vi "GeoData.vi"() -> ()   [LabVIEW 2017] (continued)
H1\n85013\t4013\tPhoenix\tAZ\tMaricopa County\tH1\n85018\t4013\tPhoenix\tAZ\tMaricopa County\tH1\n85301\t4013\tGlendale\tAZ\tMaricopa County\tH1\n85298\t4013\tGilbert\tAZ\tMaricopa County\tH1\n85338\t4013\tGoodyear\tAZ\tMaricopa County\tH1\n85353\t4013\tTolleson\tAZ\tMaricopa County\tH1\n85378\t4013\tSurprise\tAZ\tMaricopa County\tH1\n85064\t4013\tPhoenix\tAZ\tMaricopa County\tH1\n85002\t4013\tPhoenix\tAZ\tMaricopa County\tH1\n85377\t4013\tCarefree\tAZ\tMaricopa County\tH1\n85322\t4013\tArlington\tAZ\tMaricopa County\tH1\n85010\t4013\tPhoenix\tAZ\tMaricopa County\tH1\n85033\t4013\tPhoenix\tAZ\tMaricopa County\tH1\n85041\t4013\tPhoenix\tAZ\tMaricopa County\tH1\n85050\t4013\tPhoenix\tAZ\tMaricopa County\tH1\n85046\t4013\tPhoenix\tAZ\tMaricopa County\tH1\n85080\t4013\tPhoenix\tAZ\tMaricopa County\tH1\n85078\t4013\tPhoenix\tAZ\tMaricopa County\tH1\n85143\t4013\tSan tan valley\tAZ\tMaricopa County\tH1\n85209\t4013\tMesa\tAZ\tMaricopa County\tH1\n85213\t4013\tMesa\tAZ\tMaricopa County\tH1\n85250\t4013\tScottsdale\tAZ\tMaricopa County\tH1\n85261\t4013\tScottsdale\tAZ\tMaricopa County\tH1\n85007\t4013\tPhoenix\tAZ\tMaricopa County\tH1\n85012\t4013\tPhoenix\tAZ\tMaricopa County\tH1\n85015\t4013\tPhoenix\tAZ\tMaricopa County\tH1\n85306\t4013\tGlendale\tAZ\tMaricopa County\tH1\n85335\t4013\tEl mirage\tAZ\tMaricopa County\tH1\n85354\t4013\tTonopah\tAZ\tMaricopa County\tH1\n85339\t4013\tLaveen\tAZ\tMaricopa County\tH1\n85383\t4013\tPeoria\tAZ\tMaricopa County\tH1\n85274\t4013\tMesa\tAZ\tMaricopa County\tH1\n85069\t4013\tPhoenix\tAZ\tMaricopa County\tH1\n85385\t4013\tPeoria\tAZ\tMaricopa County\tH1\n85036\t4013\tPhoenix\tAZ\tMaricopa County\tH1\n85071\t4013\tPhoenix\tAZ\tMaricopa County\tH1\n85127\t4013\tChandler heights\tAZ\tMaricopa County\tH1\n85372\t4013\tSun city\tAZ\tMaricopa County\tH1\n85287\t4013\tTempe\tAZ\tMaricopa County\tH1\n86442\t4015\tBullhead city\tAZ\tMohave County\tH1\n86429\t4015\tBullhead city\tAZ\tMohave County\tH1\n86430\t4015\tBullhead city\tAZ\tMohave County\tH1\n86443\t4015\tTemple bar marina\tAZ\tMohave County\tH1\n86401\t4015\tKingman\tAZ\tMohave County\tH1\n86413\t4015\tGolden valley\tAZ\tMohave County\tH1\n86402\t4015\tKingman\tAZ\tMohave County\tH1\n86445\t4015\tWillow beach\tAZ\tMohave County\tH1\n85360\t4015\tWikieup\tAZ\tMohave County\tH1\n86404\t4015\tLake havasu city\tAZ\tMohave County\tH1\n86426\t4015\tFort mohave\tAZ\tMohave County\tH1\n86411\t4015\tHackberry\tAZ\tMohave County\tH1\n86021\t4015\tColorado city\tAZ\tMohave County\tH1\n86440\t4015\tMohave valley\tAZ\tMohave County\tH1\n86434\t4015\tPeach springs\tAZ\tMohave County\tH1\n86446\t4015\tMohave valley\tAZ\tMohave County\tH1\n86431\t4015\tChloride\tAZ\tMohave County\tH1\n86403\t4015\tLake havasu city\tAZ\tMohave County\tH1\n86406\t4015\tLake havasu city\tAZ\tMohave County\tH1\n86441\t4015\tDolan springs\tAZ\tMohave County\tH1\n86436\t4015\tTopock\tAZ\tMohave County\tH1\n86438\t4015\tYucca\tAZ\tMohave County\tH1\n86409\t4015\tKingman\tAZ\tMohave County\tH1\n86412\t4015\tHualapai\tAZ\tMohave County\tH1\n86437\t4015\tValentine\tAZ\tMohave County\tH1\n86439\t4015\tBullhead city\tAZ\tMohave County\tH1\n86432\t4015\tLittlefield\tAZ\tMohave County\tH1\n86444\t4015\tMeadview\tAZ\tMohave County\tH1\n86405\t4015\tLake havasu city\tAZ\tMohave County\tH1\n86427\t4015\tFort mohave\tAZ\tMohave County\tH1\n86433\t4015\tOatman\tAZ\tMohave County\tH1\n85942\t4017\tWoodruff\tAZ\tNavajo County\tH1\n86520\t4017\tBlue gap\tAZ\tNavajo County\tH1\n85935\t4017\tPinetop\tAZ\tNavajo County\tH1\n85901\t4017\tShow low\tAZ\tNavajo County\tH1\n86043\t4017\tSecond mesa\tAZ\tNavajo County\tH1\n85929\t4017\tLakeside\tAZ\tNavajo County\tH1\n86047\t4017\tWinslow\tAZ\tNavajo County\tH1\n86034\t4017\tKeams canyon\tAZ\tNavajo County\tH1\n85902\t4017\tShow low\tAZ\tNavajo County\tH1\n86039\t4017\tKykotsmovi village\tAZ\tNavajo County\tH1\n85926\t4017\tFort apache\tAZ\tNavajo County\tH1\n86029\t4017\tSun valley\tAZ\tNavajo County\tH1\n85928\t4017\tHeber\tAZ\tNavajo County\tH1\n86025\t4017\tHolbrook\tAZ\tNavajo County\tH1\n85933\t4017\tOvergaard\tAZ\tNavajo County\tH1\n85923\t4017\tClay springs\tAZ\tNavajo County\tH1\n85911\t4017\tCibecue\tAZ\tNavajo County\tH1\n86054\t4017\tShonto\tAZ\tNavajo County\tH1\n85937\t4017\tSnowflake\tAZ\tNavajo County\tH1\n86033\t4017\tKayenta\tAZ\tNavajo County\tH1\n86510\t4017\tPinon\tAZ\tNavajo County\tH1\n86042\t4017\tPolacca\tAZ\tNavajo County\tH1\n85939\t4017\tTaylor\tAZ\tNavajo County\tH1\n85941\t4017\tWhiteriver\tAZ\tNavajo County\tH1\n85934\t4017\tPinedale\tAZ\tNavajo County\tH1\n86031\t4017\tIndian wells\tAZ\tNavajo County\tH1\n86032\t4017\tJoseph city\tAZ\tNavajo County\tH1\n86030\t4017\tHotevilla\tAZ\tNavajo County\tH1\n85730\t4019\tTucson\tAZ\tPima County\tH1\n85740\t4019\tTucson\tAZ\tPima County\tH1\n85754\t4019\tTucson\tAZ\tPima County\tH1\n85724\t4019\tTucson\tAZ\tPima County\tH1\n85321\t4019\tAjo\tAZ\tPima County\tH1\n85736\t4019\tTucson\tAZ\tPima County\tH1\n85747\t4019\tTucson\tAZ\tPima County\tH1\n85714\t4019\tTucson\tAZ\tPima County\tH1\n85756\t4019\tTucson\tAZ\tPima County\tH1\n85658\t4019\tMarana\tAZ\tPima County\tH1\n85701\t4019\tTucson\tAZ\tPima County\tH1\n85645\t4019\tAmado\tAZ\tPima County\tH1\n85726\t4019\tTucson\tAZ\tPima County\tH1\n85743\t4019\tTucson\tAZ\tPima County\tH1\n85745\t4019\tTucson\tAZ\tPima County\tH1\n85746\t4019\tTucson\tAZ\tPima County\tH1\n85735\t4019\tTucson\tAZ\tPima County\tH1\n85733\t4019\tTucson\tAZ\tPima County\tH1\n85704\t4019\tTucson\tAZ\tPima County\tH1\n85710\t4019\tTucson\tAZ\tPima County\tH1\n85706\t4019\tTucson\tAZ\tPima County\tH1\n85734\t4019\tTucson\tAZ\tPima County\tH1\n85721\t4019\tTucson\tAZ\tPima County\tH1\n85725\t4019\tTucson\tAZ\tPima County\tH1\n85752\t4019\tTucson\tAZ\tPima County\tH1\n85601\t4019\tArivaca\tAZ\tPima County\tH1\n85633\t4019\tSasabe\tAZ\tPima County\tH1\n85719\t4019\tTucson\tAZ\tPima County\tH1\n85750\t4019\tTucson\tAZ\tPima County\tH1\n85741\t4019\tTucson\tAZ\tPima County\tH1\n85751\t4019\tTucson\tAZ\tPima County\tH1\n85702\t4019\tTucson\tAZ\tPima County\tH1\n85652\t4019\tCortaro\tAZ\tPima County\tH1\n85709\t4019\tTucson\tAZ\tPima County\tH1\n85744\t4019\tTucson\tAZ\tPima County\tH1\n85748\t4019\tTucson\tAZ\tPima County\tH1\n85715\t4019\tTucson\tAZ\tPima County\tH1\n85716\t4019\tTucson\tAZ\tPima County\tH1\n85641\t4019\tVail\tAZ\tPima County\tH1\n85653\t4019\tMarana\tAZ\tPima County\tH1\n85602\t4019\tBenson\tAZ\tPima County\tH1\n85728\t4019\tTucson\tAZ\tPima County\tH1\n85637\t4019\tSonoita\tAZ\tPima County\tH1\n85708\t4019\tTucson\tAZ\tPima County\tH1\n85634\t4019\tSells\tAZ\tPima County\tH1\n85732\t4019\tTucson\tAZ\tPima County\tH1\n85639\t4019\tTopawa\tAZ\tPima County\tH1\n85749\t4019\tTucson\tAZ\tPima County\tH1\n85713\t4019\tTucson\tAZ\tPima County\tH1\n85712\t4019\tTucson\tAZ\tPima County\tH1\n85757\t4019\tTucson\tAZ\tPima County\tH1\n85711\t4019\tTucson\tAZ\tPima County\tH1\n85622\t4019\tGreen valley\tAZ\tPima County\tH1\n85703\t4019\tTucson\tAZ\tPima County\tH1\n85619\t4019\tMount lemmon\tAZ\tPima County\tH1\n85654\t4019\tRillito\tAZ\tPima County\tH1\n85718\t4019\tTucson\tAZ\tPima County\tH1\n85755\t4019\tTucson\tAZ\tPima County\tH1\n85742\t4019\tTucson\tAZ\tPima County\tH1\n85707\t4019\tTucson\tAZ\tPima County\tH1\n85738\t4019\tCatalina\tAZ\tPima County\tH1\n85731\t4019\tTucson\tAZ\tPima County\tH1\n85723\t4019\tTucson\tAZ\tPima County\tH1\n85737\t4019\tTucson\tAZ\tPima County\tH1\n85739\t4019\tTucson\tAZ\tPima County\tH1\n85614\t4019\tGreen valley\tAZ\tPima County\tH1\n85705\t4019\tTucson\tAZ\tPima County\tH1\n85629\t4019\tSahuarita\tAZ\tPima County\tH1\n85611\t4019\tElgin\tAZ\tPima County\tH1\n85717\t4019\tTucson\tAZ\tPima County\tH1\n85341\t4019\tLukeville\tAZ\tPima County\tH1\n85117\t4021\tApache junction\tAZ\tPinal County\tH1\n85178\t4021\tApache junction\tAZ\tPinal County\tH1\n85192\t4021\tWinkelman\tAZ\tPinal County\tH1\n85191\t4021\tValley farms\tAZ\tPinal County\tH1\n85119\t4021\tApache junction\tAZ\tPinal County\tH1\n85139\t4021\tMaricopa\tAZ\tPinal County\tH1\n85194\t4021\tCasa grande\tAZ\tPinal County\tH1\n85120\t4021\tApache junction\tAZ\tPinal County\tH1\n85173\t4021\tSuperior\tAZ\tPinal County\tH1\n85658\t4021\tMarana\tAZ\tPinal County\tH1\n85193\t4021\tCasa grande\tAZ\tPinal County\tH1\n85128\t4021\tCoolidge\tAZ\tPinal County\tH1\n85140\t4021\tSan tan valley\tAZ\tPinal County\tH1\n85618\t4021\tMammoth\tAZ\tPinal County\tH1\n85631\t4021\tSan manuel\tAZ\tPinal County\tH1\n85145\t4021\tRed rock\tAZ\tPinal County\tH1\n85137\t4021\tKearny\tAZ\tPinal County\tH1\n85122\t4021\tCasa grande\tAZ\tPinal County\tH1\n85142\t4021\tQueen creek\tAZ\tPinal County\tH1\n85623\t4021\tOracle\tAZ\tPinal County\tH1\n85172\t4021\tStanfield\tAZ\tPinal County\tH1\n85130\t4021\tCasa grande\tAZ\tPinal County\tH1\n85653\t4021\tMarana\tAZ\tPinal County\tH1\n85602\t4021\tBenson\tAZ\tPinal County\tH1\n85141\t4021\tPicacho\tAZ\tPinal County\tH1\n85118\t4021\tGold canyon\tAZ\tPinal County\tH1\n85138\t4021\tMaricopa\tAZ\tPinal County\tH1\n85132\t4021\tFlorence\tAZ\tPinal County\tH1\n85212\t4021\tMesa\tAZ\tPinal County\tH1\n85248\t4021\tChandler\tAZ\tPinal County\tH1\n85539\t4021\tMiami\tAZ\tPinal County\tH1\n85143\t4021\tSan tan valley\tAZ\tPinal County\tH1\n85131\t4021\tEloy\tAZ\tPinal County\tH1\n85739\t4021\tTucson\tAZ\tPinal County\tH1\n85640\t4023\tTumacacori\tAZ\tSanta Cruz County\tH1\n85645\t4023\tAmado\tAZ\tSanta Cruz County\tH1\n85621\t4023\tNogales\tAZ\tSanta Cruz County\tH1\n85628\t4023\tNogales\tAZ\tSanta Cruz County\tH1\n85637\t4023\tSonoita\tAZ\tSanta Cruz County\tH1\n85624\t4023\tPatagonia\tAZ\tSanta Cruz County\tH1\n85648\t4023\tRio rico\tAZ\tSanta Cruz County\tH1\n85646\t4023\tTubac\tAZ\tSanta Cruz County\tH1\n85614\t4023\tGreen valley\tAZ\tSanta Cruz County\tH1\n85611\t4023\tElgin\tAZ\tSanta Cruz County\tH1\n86314\t4025\tPrescott valley\tAZ\tYavapai County\tH1\n86333\t4025\tMayer\tAZ\tYavapai County\tH1\n86313\t4025\tPrescott\tAZ\tYavapai County\tH1\n86303\t4025\tPrescott\tAZ\tYavapai County\tH1\n86315\t4025\tPrescott valley\tAZ\tYavapai County\tH1\n86351\t4025\tSedona\tAZ\tYavapai County\tH1\n86327\t4025\tDewey\tAZ\tYavapai County\tH1\n86336\t4025\tSedona\tAZ\tYavapai County\tH1\n86332\t4025\tKirkland\tAZ\tYavapai County\tH1\n86334\t4025\tPaulden\tAZ\tYavapai County\tH1\n86331\t4025\tJerome\tAZ\tYavapai County\tH1\n86301\t4025\tPrescott\tAZ\tYavapai County\tH1\n86305\t4025\tPrescott\tAZ\tYavapai County\tH1\n86323\t4025\tChino valley\tAZ\tYavapai County\tH1\n86325\t4025\tCornville\tAZ\tYavapai County\tH1\n86320\t4025\tAsh fork\tAZ\tYavapai County\tH1\n86338\t4025\tSkull valley\tAZ\tYavapai County\tH1\n86343\t4025\tCrown king\tAZ\tYavapai County\tH1\n86342\t4025\tLake montezuma\tAZ\tYavapai County\tH1\n85390\t4025\tWickenburg\tAZ\tYavapai County\tH1\n85342\t4025\tMorristown\tAZ\tYavapai County\tH1\n86335\t4025\tRimrock\tAZ\tYavapai County\tH1\n86312\t4025\tPrescott valley\tAZ\tYavapai County\tH1\n86304\t4025\tPrescott\tAZ\tYavapai County\tH1\n85324\t4025\tBlack canyon city\tAZ\tYavapai County\tH1\n86326\t4025\tCottonwood\tAZ\tYavapai County\tH1\n86337\t4025\tSeligman\tAZ\tYavapai County\tH1\n85332\t4025\tCongress\tAZ\tYavapai County\tH1\n86329\t4025\tHumboldt\tAZ\tYavapai County\tH1\n86322\t4025\tCamp verde\tAZ\tYavapai County\tH1\n86046\t4025\tWilliams\tAZ\tYavapai County\tH1\n86302\t4025\tPrescott\tAZ\tYavapai County\tH1\n86340\t4025\tSedona\tAZ\tYavapai County\tH1\n86321\t4025\tBagdad\tAZ\tYavapai County\tH1\n86324\t4025\tClarkdale\tAZ\tYavapai County\tH1\n85362\t4025\tYarnell\tAZ\tYavapai County\tH1\n85364\t4027\tYuma\tAZ\tYuma County\tH1\n85366\t4027\tYuma\tAZ\tYuma County\tH1\n85347\t4027\tRoll\tAZ\tYuma County\tH1\n85333\t4027\tDateland\tAZ\tYuma County\tH1\n85367\t4027\tYuma\tAZ\tYuma County\tH1\n85349\t4027\tSan luis\tAZ\tYuma County\tH1\n85356\t4027\tWellton\tAZ\tYuma County\tH1\n85350\t4027\tSomerton\tAZ\tYuma County\tH1\n85352\t4027\tTacna\tAZ\tYuma County\tH1\n85365\t4027\tYuma\tAZ\tYuma County\tH1\n85336\t4027\tGadsden\tAZ\tYuma County\tH1\n72073\t5001\tHumphrey\tAR\tArkansas County\tH1\n72004\t5001\tAltheimer\tAR\tArkansas County\tH1\n72134\t5001\tRoe\tAR\tArkansas County\tH1\n72055\t5001\tGillett\tAR\tArkansas County\tH1\n72048\t5001\tEthel\tAR\tArkansas County\tH1\n72042\t5001\tDe witt\tAR\tArkansas County\tH1\n72166\t5001\tTichnor\tAR\tArkansas County\tH1\n72140\t5001\tSaint charles\tAR\tArkansas County\tH1\n72038\t5001\tCrocketts bluff\tAR\tArkansas County\tH1\n72160\t5001\tStuttgart\tAR\tArkansas County\tH1\n72026\t5001\tCasscoe\tAR\tArkansas County\tH1\n72003\t5001\tAlmyra\tAR\tArkansas County\tH1\n71663\t5003\tPortland\tAR\tAshley County\tH1\n71640\t5003\tEudora\tAR\tAshley County\tH1\n71661\t5003\tParkdale\tAR\tAshley County\tH1\n71646\t5003\tHamburg\tAR\tAshley County\tH1\n71635\t5003\tCrossett\tAR\tAshley County\tH1\n71638\t5003\tDermott\tAR\tAshley County\tH1\n71642\t5003\tFountain hill\tAR\tAshley County\tH1\n71658\t5003\tMontrose\tAR\tAshley County\tH1\n71676\t5003\tWilmot\tAR\tAshley County\tH1\n72531\t5005\tElizabeth\tAR\tBaxter County\tH1\n72617\t5005\tBig flat\tAR\tBaxter County\tH1\n72538\t5005\tGepp\tAR\tBaxter County\tH1\n72635\t5005\tGassville\tAR\tBaxter County\tH1\n72642\t5005\tLakeview\tAR\tBaxter County\tH1\n72544\t5005\tHenderson\tAR\tBaxter County\tH1\n72626\t5005\tCotter\tAR\tBaxter County\tH1\n72651\t5005\tMidway\tAR\tBaxter County\tH1\n72623\t5005\tClarkridge\tAR\tBaxter County\tH1\n72653\t5005\tMountain home\tAR\tBaxter County\tH1\n72658\t5005\tNorfork\tAR\tBaxter County\tH1\n72519\t5005\tCalico rock\tAR\tBaxter County\tH1\n72537\t5005\tGamaliel\tAR\tBaxter County\tH1\n72654\t5005\tMountain home\tAR\tBaxter County\tH1\n72659\t5005\tNorfork\tAR\tBaxter County\tH1\n72732\t5007\tGarfield\tAR\tBenton County\tH1\n72758\t5007\tRogers\tAR\tBenton County\tH1\n72761\t5007\tSiloam springs\tAR\tBenton County\tH1\n72764\t5007\tSpringdale\tAR\tBenton County\tH1\n72751\t5007\tPea ridge\tAR\tBenton County\tH1\n72733\t5007\tGateway\tAR\tBenton County\tH1\n72745\t5007\tLowell\tAR\tBenton County\tH1\n72768\t5007\tSulphur springs\tAR\tBenton County\tH1\n72739\t5007\tHiwasse\tAR\tBenton County\tH1\n72712\t5007\tBentonville\tAR\tBenton County\tH1\n72734\t5007\tGentry\tAR\tBenton County\tH1\n72756\t5007\tRogers\tAR\tBenton County\tH1\n72722\t5007\tDecatur\tAR\tBenton County\tH1\n72716\t5007\tBentonville\tAR\tBenton County\tH1\n72704\t5007\tFayetteville\tAR\tBenton County\tH1\n72718\t5007\tCave springs\tAR\tBenton County\tH1\n72714\t5007\tBella vista\tAR\tBenton County\tH1\n72736\t5007\tGravette\tAR\tBenton County\tH1\n72747\t5007\tMaysville\tAR\tBenton County\tH1\n72757\t5007\tRogers\tAR\tBenton County\tH1\n72738\t5007\tHindsville\tAR\tBenton County\tH1\n72762\t5007\tSpringdale\tAR\tBenton County\tH1\n72719\t5007\tCenterton\tAR\tBenton County\tH1\n72715\t5007\tBella vista\tAR\tBenton County\tH1\n72711\t5007\tAvoca\tAR\tBenton County\tH1\n72685\t5009\tWestern grove\tAR\tBoone County\tH1\n72601\t5009\tHarrison\tAR\tBoone County\tH1\n72662\t5009\tOmaha\tAR\tBoone County\tH1\n72615\t5009\tBergman\tAR\tBoone County\tH1\n72633\t5009\tEverton\tAR\tBoone County\tH1\n72611\t5009\tAlpena\tAR\tBoone County\tH1\n72602\t5009\tHarrison\tAR\tBoone County\tH1\n72687\t5009\tYellville\tAR\tBoone County\tH1\n72644\t5009\tLead hill\tAR\tBoone County\tH1\n72682\t5009\tValley springs\tAR\tBoone County\tH1\n71651\t5011\tJersey\tAR\tBradley County\tH1\n71647\t5011\tHermitage\tAR\tBradley County\tH1\n71671\t5011\tWarren\tAR\tBradley County\tH1\n71675\t5011\tWilmar\tAR\tBradley County\tH1\n71631\t5011\tBanks\tAR\tBradley County\tH1\n71660\t5011\tNew edinburg\tAR\tBradley County\tH1\n71701\t5013\tCamden\tAR\tCalhoun County\tH1\n71744\t5013\tHampton\tAR\tCalhoun County\tH1\n71720\t5013\tBearden\tAR\tCalhoun County\tH1\n71745\t5013\tHarrell\tAR\tCalhoun County\tH1\n71742\t5013\tFordyce\tAR\tCalhoun County\tH1\n71766\t5013\tThornton\tAR\tCalhoun County\tH1\n72740\t5015\tHuntsville\tAR\tCarroll County\tH1\n72632\t5015\tEureka springs\tAR\tCarroll County\tH1\n72631\t5015\tEureka springs\tAR\tCarroll County\tH1\n72601\t5015\tHarrison\tAR\tCarroll County\tH1\n72624\t5015\tCompton\tAR\tCarroll County\tH1\n72662\t5015\tOmaha\tAR\tCarroll County\tH1\n72660\t5015\tOak grove\tAR\tCarroll County\tH1\n72638\t5015\tGreen forest\tAR\tCarroll County\tH1\n72611\t5015\tAlpena\tAR\tCarroll County\tH1\n72616\t5015\tBerryville\tAR\tCarroll County\tH1\n72613\t5015\tBeaver\tAR\tCarroll County\tH1\n71653\t5017\tLake village\tAR\tChicot County\tH1\n71663\t5017\tPortland\tAR\tChicot County\tH1\n71640\t5017\tEudora\tAR\tChicot County\tH1\n71661\t5017\tParkdale\tAR\tChicot County\tH1\n71638\t5017\tDermott\tAR\tChicot County\tH1\n71676\t5017\tWilmot\tAR\tChicot County\tH1\n71728\t5019\tCurtis\tAR\tClark County\tH1\n71743\t5019\tGurdon\tAR\tClark County\tH1\n71962\t5019\tOkolona\tAR\tClark County\tH1\n71763\t5019\tSparkman\tAR\tClark County\tH1\n71721\t5019\tBeirne\tAR\tClark County\tH1\n71998\t5019\tArkadelphia\tAR\tClark County\tH1\n71921\t5019\tAmity\tAR\tClark County\tH1\n71929\t5019\tBismarck\tAR\tClark County\tH1\n71772\t5019\tWhelen springs\tAR\tClark County\tH1\n71999\t5019\tArkadelphia\tAR\tClark County\tH1\n71923\t5019\tArkadelphia\tAR\tClark County\tH1\n72430\t5021\tGreenway\tAR\tClay County\tH1\n72436\t5021\tLafe\tAR\tClay County\tH1\n72413\t5021\tBiggers\tAR\tClay County\tH1\n72453\t5021\tPeach orchard\tAR\tClay County\tH1\n72435\t5021\tKnobel\tAR\tClay County\tH1\n72461\t5021\tRector\tAR\tClay County\tH1\n72464\t5021\tSaint francis\tAR\tClay County\tH1\n72456\t5021\tPollard\tAR\tClay County\tH1\n72424\t5021\tDatto\tAR\tClay County\tH1\n72470\t5021\tSuccess\tAR\tClay County\tH1\n72441\t5021\tMc dougal\tAR\tClay County\tH1\n72454\t5021\tPiggott\tAR\tClay County\tH1\n72422\t5021\tCorning\tAR\tClay County\tH1\n72425\t5021\tDelaplaine\tAR\tClay County\tH1\n72153\t5023\tShirley\tAR\tCleburne County\tH1\n72581\t5023\tTumbling shoals\tAR\tCleburne County\tH1\n72044\t5023\tEdgemont\tAR\tCleburne County\tH1\n72179\t5023\tWilburn\tAR\tCleburne County\tH1\n72121\t5023\tPangburn\tAR\tCleburne County\tH1\n72067\t5023\tHigden\tAR\tCleburne County\tH1\n72131\t5023\tQuitman\tAR\tCleburne County\tH1\n72143\t5023\tSearcy\tAR\tCleburne County\tH1\n72530\t5023\tDrasco\tAR\tCleburne County\tH1\n72534\t5023\tFloral\tAR\tCleburne County\tH1\n72523\t5023\tConcord\tAR\tCleburne County\tH1\n72634\t5023\tFlippin\tAR\tCleburne County\tH1\n72550\t5023\tLocust grove\tAR\tCleburne County\tH1\n72546\t5023\tIda\tAR\tCleburne County\tH1\n72543\t5023\tHeber springs\tAR\tCleburne County\tH1\n72130\t5023\tPrim\tAR\tCleburne County\tH1\n72088\t5023\tFairfield bay\tAR\tCleburne County\tH1\n72137\t5023\tRose bud\tAR\tCleburne County\tH1\n72545\t5023\tHeber springs\tAR\tCleburne County\tH1\n72057\t5025\tGrapevine\tAR\tCleveland County\tH1\n71603\t5025\tPine bluff\tAR\tCleveland County\tH1\n71671\t5025\tWarren\tAR\tCleveland County\tH1\n71665\t5025\tRison\tAR\tCleveland County\tH1\n71667\t5025\tStar city\tAR\tCleveland County\tH1\n71652\t5025\tKingsland\tAR\tCleveland County\tH1\n71660\t5025\tNew edinburg\tAR\tCleveland County\tH1\n71861\t5027\tTaylor\tAR\tColumbia County\tH1\n71764\t5027\tStephens\tAR\tColumbia County\tH1\n71753\t5027\tMagnolia\tAR\tColumbia County\tH1\n71754\t5027\tMagnolia\tAR\tColumbia County\tH1\n71770\t5027\tWaldo\tAR\tColumbia County\tH1\n71752\t5027\tMc neil\tAR\tColumbia County\tH1\n71860\t5027\tStamps\tAR\tColumbia County\tH1\n71740\t5027\tEmerson\tAR\tColumbia County\tH1\n72001\t5029\tAdona\tAR\tConway County\tH1\n72013\t5029\tBee branch\tAR\tConway County\tH1\n72107\t5029\tMenifee\tAR\tConway County\tH1\n72030\t5029\tCleveland\tAR\tConway County\tH1\n72027\t5029\tCenter ridge\tAR\tConway County\tH1\n72156\t5029\tSolgohachia\tAR\tConway County\tH1\n72125\t5029\tPerry\tAR\tConway County\tH1\n72110\t5029\tMorrilton\tAR\tConway County\tH1\n72823\t5029\tAtkins\tAR\tConway County\tH1\n72127\t5029\tPlumerville\tAR\tConway County\tH1\n72025\t5029\tCasa\tAR\tConway County\tH1\n72080\t5029\tJerusalem\tAR\tConway County\tH1\n72063\t5029\tHattieville\tAR\tConway County\tH1\n72031\t5029\tClinton\tAR\tConway County\tH1\n72157\t5029\tSpringfield\tAR\tConway County\tH1\n72421\t5031\tCash\tAR\tCraighead County\tH1\n72402\t5031\tJonesboro\tAR\tCraighead County\tH1\n72437\t5031\tLake city\tAR\tCraighead County\tH1\n72416\t5031\tBono\tAR\tCraighead County\tH1\n72447\t5031\tMonette\tAR\tCraighead County\tH1\n72427\t5031\tEgypt\tAR\tCraighead County\tH1\n72403\t5031\tJonesboro\tAR\tCraighead County\tH1\n72438\t5031\tLeachville\tAR\tCraighead County\tH1\n72414\t5031\tBlack oak\tAR\tCraighead County\tH1\n72472\t5031\tTrumann\tAR\tCraighead County\tH1\n72404\t5031\tJonesboro\tAR\tCraighead County\tH1\n72411\t5031\tBay\tAR\tCraighead County\tH1\n72401\t5031\tJonesboro\tAR\tCraighead County\tH1\n72476\t5031\tWalnut ridge\tAR\tCraighead County\tH1\n72419\t5031\tCaraway\tAR\tCraighead County\tH1\n72467\t5031\tState university\tAR\tCraighead County\tH1\n72450\t5031\tParagould\tAR\tCraighead County\tH1\n72417\t5031\tBrookland\tAR\tCraighead County\tH1\n72479\t5031\tWeiner\tAR\tCraighead County\tH1\n72956\t5033\tVan buren\tAR\tCrawford County\tH1\n72955\t5033\tUniontown\tAR\tCrawford County\tH1\n72952\t5033\tRudy\tAR\tCrawford County\tH1\n72935\t5033\tDyer\tAR\tCrawford County\tH1\n72932\t5033\tCedarville\tAR\tCrawford County\tH1\n72959\t5033\tWinslow\tAR\tCrawford County\tH1\n72948\t5033\tNatural dam\tAR\tCrawford County\tH1\n72946\t5033\tMountainburg\tAR\tCrawford County\tH1\n72774\t5033\tWest fork\tAR\tCrawford County\tH1\n72957\t5033\tVan buren\tAR\tCrawford County\tH1\n72921\t5033\tAlma\tAR\tCrawford County\tH1\n72934\t5033\tChester\tAR\tCrawford County\tH1\n72947\t5033\tMulberry\tAR\tCrawford County\tH1\n72327\t5035\tCrawfordsville\tAR\tCrittenden County\tH1\n72301\t5035\tWest memphis\tAR\tCrittenden County\tH1\n72331\t5035\tEarle\tAR\tCrittenden County\tH1\n72325\t5035\tClarkedale\tAR\tCrittenden County\tH1\n72332\t5035\tEdmondson\tAR\tCrittenden County\tH1\n72348\t5035\tHughes\tAR\tCrittenden County\tH1\n72339\t5035\tGilmore\tAR\tCrittenden County\tH1\n72364\t5035\tMarion\tAR\tCrittenden County\tH1\n72386\t5035\tTyronza\tAR\tCrittenden County\tH1\n72376\t5035\tProctor\tAR\tCrittenden County\tH1\n72384\t5035\tTurrell\tAR\tCrittenden County\tH1\n72396\t5037\tWynne\tAR\tCross County\tH1\n72331\t5037\tEarle\tAR\tCross County\tH1\n72373\t5037\tParkin\tAR\tCross County\tH1\n72346\t5037\tHeth\tAR\tCross County\tH1\n72347\t5037\tHickory ridge\tAR\tCross County\tH1\n72326\t5037\tColt\tAR\tCross County\tH1\n72101\t5037\tMc crory\tAR\tCross County\tH1\n72324\t5037\tCherry valley\tAR\tCross County\tH1\n72387\t5037\tVanndale\tAR\tCross County\tH1\n71725\t5039\tCarthage\tAR\tDallas County\tH1\n71720\t5039\tBearden\tAR\tDallas County\tH1\n71763\t5039\tSparkman\tAR\tDallas County\tH1\n72084\t5039\tLeola\tAR\tDallas County\tH1\n71742\t5039\tFordyce\tAR\tDallas County\tH1\n71652\t5039\tKingsland\tAR\tDallas County\tH1\n71748\t5039\tIvan\tAR\tDallas County\tH1\n71923\t5039\tArkadelphia\tAR\tDallas County\tH1\n71662\t5041\tPickens\tAR\tDesha County\tH1\n72379\t5041\tSnow lake\tAR\tDesha County\tH1\n71639\t5041\tDumas\tAR\tDesha County\tH1\n71638\t5041\tDermott\tAR\tDesha County\tH1\n71654\t5041\tMc gehee\tAR\tDesha County\tH1\n71670\t5041\tTillar\tAR\tDesha County\tH1\n71674\t5041\tWatson\tAR\tDesha County\tH1\n71643\t5041\tGould\tAR\tDesha County\tH1\n71630\t5041\tArkansas city\tAR\tDesha County\tH1\n71677\t5043\tWinchester\tAR\tDrew County\tH1\n71655\t5043\tMonticello\tAR\tDrew County\tH1\n71646\t5043\tHamburg\tAR\tDrew County\tH1\n71638\t5043\tDermott\tAR\tDrew County\tH1\n71675\t5043\tWilmar\tAR\tDrew County\tH1\n71670\t5043\tTillar\tAR\tDrew County\tH1\n71642\t5043\tFountain hill\tAR\tDrew County\tH1\n71658\t5043\tMontrose\tAR\tDrew County\tH1\n72039\t5045\tDamascus\tAR\tFaulkner County\tH1\n72033\t5045\tConway\tAR\tFaulkner County\tH1\n72023\t5045\tCabot\tAR\tFaulkner County\tH1\n72131\t5045\tQuitman\tAR\tFaulkner County\tH1\n72120\t5045\tSherwood\tAR\tFaulkner County\tH1\n72181\t5045\tWooster\tAR\tFaulkner County\tH1\n72034\t5045\tConway\tAR\tFaulkner County\tH1\n72106\t5045\tMayflower\tAR\tFaulkner County\tH1\n72061\t5045\tGuy\tAR\tFaulkner County\tH1\n72076\t5045\tJacksonville\tAR\tFaulkner County\tH1\n72058\t5045\tGreenbrier\tAR\tFaulkner County\tH1\n72035\t5045\tConway\tAR\tFaulkner County\tH1\n72173\t5045\tVilonia\tAR\tFaulkner County\tH1\n72111\t5045\tMount vernon\tAR\tFaulkner County\tH1\n72016\t5045\tBigelow\tAR\tFaulkner County\tH1\n72047\t5045\tEnola\tAR\tFaulkner County\tH1\n72032\t5045\tConway\tAR\tFaulkner County\tH1\n72933\t5047\tCharleston\tAR\tFranklin County\tH1\n72928\t5047\tBranch\tAR\tFranklin County\tH1\n72821\t5047\tAltus\tAR\tFranklin County\tH1\n72943\t5047\tMagazine\tAR\tFranklin County\tH1\n72820\t5047\tAlix\tAR\tFranklin County\tH1\n72951\t5047\tRatcliff\tAR\tFranklin County\tH1\n72959\t5047\tWinslow\tAR\tFranklin County\tH1\n72721\t5047\tCombs\tAR\tFranklin County\tH1\n72946\t5047\tMountainburg\tAR\tFranklin County\tH1\n72930\t5047\tCecil\tAR\tFranklin County\tH1\n72949\t5047\tOzark\tAR\tFranklin County\tH1\n72855\t5047\tParis\tAR\tFranklin County\tH1\n72947\t5047\tMulberry\tAR\tFranklin County\tH1\n72542\t5049\tHardy\tAR\tFulton County\tH1\n72531\t5049\tElizabeth\tAR\tFulton County\tH1\n72528\t5049\tDolph\tAR\tFulton County\tH1\n72539\t5049\tGlencoe\tAR\tFulton County\tH1\n72538\t5049\tGepp\tAR\tFulton County\tH1\n72554\t5049\tMammoth spring\tAR\tFulton County\tH1\n72515\t5049\tBexar\tAR\tFulton County\tH1\n72529\t5049\tCherokee village\tAR\tFulton County\tH1\n72520\t5049\tCamp\tAR\tFulton County\tH1\n72578\t5049\tSturkie\tAR\tFulton County\tH1\n72576\t5049\tSalem\tAR\tFulton County\tH1\n72513\t5049\tAsh flat\tAR\tFulton County\tH1\n72583\t5049\tViola\tAR\tFulton County\tH1\n72512\t5049\tHorseshoe bend\tAR\tFulton County\tH1\n72566\t5049\tPineville\tAR\tFulton County\tH1\n71933\t5051\tBonnerdale\tAR\tGarland County\tH1\n72104\t5051\tMalvern\tAR\tGarland County\tH1\n71964\t5051\tPearcy\tAR\tGarland County\tH1\n71910\t5051\tHot springs village\tAR\tGarland County\tH1\n72941\t5051\tLavaca\tAR\tGarland County\tH1\n71902\t5051\tHot springs national park\tAR\tGarland County\tH1\n71901\t5051\tHot springs national park\tAR\tGarland County\tH1\n71909\t5051\tHot springs village\tAR\tGarland County\tH1\n72087\t5051\tLonsdale\tAR\tGarland County\tH1\n71914\t5051\tHot springs national park\tAR\tGarland County\tH1\n71956\t5051\tMountain pine\tAR\tGarland County\tH1\n71949\t5051\tJessieville\tAR\tGarland County\tH1\n71913\t5051\tHot springs national park\tAR\tGarland County\tH1\n71903\t5051\tHot springs national park\tAR\tGarland County\tH1\n71968\t5051\tRoyal\tAR\tGarland County\tH1\n72057\t5053\tGrapevine\tAR\tGrant County\tH1\n72129\t5053\tPrattsville\tAR\tGrant County\tH1\n71603\t5053\tPine bluff\tAR\tGrant County\tH1\n72065\t5053\tHensley\tAR\tGrant County\tH1\n72079\t5053\tJefferson\tAR\tGrant County\tH1\n71602\t5053\tWhite hall\tAR\tGrant County\tH1\n72104\t5053\tMalvern\tAR\tGrant County\tH1\n72084\t5053\tLeola\tAR\tGrant County\tH1\n72167\t5053\tTraskwood\tAR\tGrant County\tH1\n72128\t5053\tPoyen\tAR\tGrant County\tH1\n72150\t5053\tSheridan\tAR\tGrant County\tH1\n72015\t5053\tBenton\tAR\tGrant County\tH1\n72011\t5053\tBauxite\tAR\tGrant County\tH1\n72132\t5053\tRedfield\tAR\tGrant County\tH1\n72436\t5055\tLafe\tAR\tGreene County\tH1\n72453\t5055\tPeach orchard\tAR\tGreene County\tH1\n72416\t5055\tBono\tAR\tGreene County\tH1\n72435\t5055\tKnobel\tAR\tGreene County\tH1\n72461\t5055\tRector\tAR\tGreene County\tH1\n72412\t5055\tBeech grove\tAR\tGreene County\tH1\n72401\t5055\tJonesboro\tAR\tGreene County\tH1\n72443\t5055\tMarmaduke\tAR\tGreene County\tH1\n72451\t5055\tParagould\tAR\tGreene County\tH1\n72474\t5055\tWalcott\tAR\tGreene County\tH1\n72450\t5055\tParagould\tAR\tGreene County\tH1\n72417\t5055\tBrookland\tAR\tGreene County\tH1\n72425\t5055\tDelaplaine\tAR\tGreene County\tH1\n71862\t5057\tWashington\tAR\tHempstead County\tH1\n71855\t5057\tOzan\tAR\tHempstead County\tH1\n71847\t5057\tMc caskill\tAR\tHempstead County\tH1\n71857\t5057\tPrescott\tAR\tHempstead County\tH1\n71838\t5057\tFulton\tAR\tHempstead County\tH1\n71825\t5057\tBlevins\tAR\tHempstead County\tH1\n71831\t5057\tColumbus\tAR\tHempstead County\tH1\n71801\t5057\tHope\tAR\tHempstead County\tH1\n71835\t5057\tEmmet\tAR\tHempstead County\tH1\n71852\t5057\tNashville\tAR\tHempstead County\tH1\n71822\t5057\tAshdown\tAR\tHempstead County\tH1\n71859\t5057\tSaratoga\tAR\tHempstead County\tH1\n71933\t5059\tBonnerdale\tAR\tHot Spring County\tH1\n71941\t5059\tDonaldson\tAR\tHot Spring County\tH1\n71943\t5059\tGlenwood\tAR\tHot Spring County\tH1\n72104\t5059\tMalvern\tAR\tHot Spring County\tH1\n72084\t5059\tLeola\tAR\tHot Spring County\tH1\n71964\t5059\tPearcy\tAR\tHot Spring County\tH1\n72167\t5059\tTraskwood\tAR\tHot Spring County\tH1\n72128\t5059\tPoyen\tAR\tHot Spring County\tH1\n71921\t5059\tAmity\tAR\tHot Spring County\tH1\n71929\t5059\tBismarck\tAR\tHot Spring County\tH1\n71901\t5059\tHot springs national park\tAR\tHot Spring County\tH1\n71923\t5059\tArkadelphia\tAR\tHot Spring County\tH1\n71942\t5059\tFriendship\tAR\tHot Spring County\tH1\n71913\t5059\tHot springs national park\tAR\tHot Spring County\tH1\n71971\t5061\tUmpire\tAR\tHoward County\tH1\n71833\t5061\tDierks\tAR\tHoward County\tH1\n71973\t5061\tWickes\tAR\tHoward County\tH1\n71851\t5061\tMineral springs\tAR\tHoward County\tH1\n71831\t5061\tColumbus\tAR\tHoward County\tH1\n71959\t5061\tNewhope\tAR\tHoward County\tH1\n71852\t5061\tNashville\tAR\tHoward County\tH1\n71859\t5061\tSaratoga\tAR\tHoward County\tH1\n72112\t5063\tNewport\tAR\tIndependence County\tH1\n72524\t5063\tCord\tAR\tIndependence County\tH1\n72568\t5063\tPleasant plains\tAR\tIndependence County\tH1\n72527\t5063\tDesha\tAR\tIndependence County\tH1\n72081\t5063\tJudsonia\tAR\tIndependence County\tH1\n72521\t5063\tCave city\tAR\tIndependence County\tH1\n72526\t5063\tCushman\tAR\tIndependence County\tH1\n72534\t5063\tFloral\tAR\tIndependence County\tH1\n72562\t5063\tNewark\tAR\tIndependence County\tH1\n72523\t5063\tConcord\tAR\tIndependence County\tH1\n72550\t5063\tLocust grove\tAR\tIndependence County\tH1\n72564\t5063\tOil trough\tAR\tIndependence County\tH1\n72572\t5063\tSaffell\tAR\tIndependence County\tH1\n72165\t5063\tThida\tAR\tIndependence County\tH1\n72575\t5063\tSalado\tAR\tIndependence County\tH1\n72020\t5063\tBradford\tAR\tIndependence County\tH1\n72501\t5063\tBatesville\tAR\tIndependence County\tH1\n72579\t5063\tSulphur rock\tAR\tIndependence County\tH1\n72571\t5063\tRosie\tAR\tIndependence County\tH1\n72522\t5063\tCharlotte\tAR\tIndependence County\tH1\n72553\t5063\tMagness\tAR\tIndependence County\tH1\n72561\t5065\tMount pleasant\tAR\tIzard County\tH1\n72528\t5065\tDolph\tAR\tIzard County\tH1\n72584\t5065\tViolet hill\tAR\tIzard County\tH1\n72556\t5065\tMelbourne\tAR\tIzard County\tH1\n72517\t5065\tBrockwell\tAR\tIzard County\tH1\n72532\t5065\tEvening shade\tAR\tIzard County\tH1\n72540\t5065\tGuion\tAR\tIzard County\tH1\n72587\t5065\tWiseman\tAR\tIzard County\tH1\n72501\t5065\tBatesville\tAR\tIzard County\tH1\n72573\t5065\tSage\tAR\tIzard County\tH1\n72585\t5065\tWideman\tAR\tIzard County\tH1\n72513\t5065\tAsh flat\tAR\tIzard County\tH1\n72536\t5065\tFranklin\tAR\tIzard County\tH1\n72519\t5065\tCalico rock\tAR\tIzard County\tH1\n72512\t5065\tHorseshoe bend\tAR\tIzard County\tH1\n72560\t5065\tMountain view\tAR\tIzard County\tH1\n72566\t5065\tPineville\tAR\tIzard County\tH1\n72565\t5065\tOxford\tAR\tIzard County\tH1\n72577\t5065\tSidney\tAR\tIzard County\tH1\n72112\t5067\tNewport\tAR\tJackson County\tH1\n72431\t5067\tGrubbs\tAR\tJackson County\tH1\n72169\t5067\tTupelo\tAR\tJackson County\tH1\n72043\t5067\tDiaz\tAR\tJackson County\tH1\n72473\t5067\tTuckerman\tAR\tJackson County\tH1\n72347\t5067\tHickory ridge\tAR\tJackson County\tH1\n72471\t5067\tSwifton\tAR\tJackson County\tH1\n72005\t5067\tAmagon\tAR\tJackson County\tH1\n72014\t5067\tBeedeville\tAR\tJackson County\tH1\n72020\t5067\tBradford\tAR\tJackson County\tH1\n72101\t5067\tMc crory\tAR\tJackson County\tH1\n72479\t5067\tWeiner\tAR\tJackson County\tH1\n72075\t5067\tJacksonport\tAR\tJackson County\tH1\n72073\t5069\tHumphrey\tAR\tJefferson County\tH1\n72133\t5069\tReydell\tAR\tJefferson County\tH1\n71603\t5069\tPine bluff\tAR\tJefferson County\tH1\n72004\t5069\tAltheimer\tAR\tJefferson County\tH1\n72079\t5069\tJefferson\tAR\tJefferson County\tH1\n71602\t5069\tWhite hall\tAR\tJefferson County\tH1\n72072\t5069\tHumnoke\tAR\tJefferson County\tH1\n71659\t5069\tMoscow\tAR\tJefferson County\tH1\n72046\t5069\tEngland\tAR\tJefferson County\tH1\n72182\t5069\tWright\tAR\tJefferson County\tH1\n71665\t5069\tRison\tAR\tJefferson County\tH1\n71601\t5069\tPine bluff\tAR\tJefferson County\tH1\n72150\t5069\tSheridan\tAR\tJefferson County\tH1\n72160\t5069\tStuttgart\tAR\tJefferson County\tH1\n72175\t5069\tWabbaseka\tAR\tJefferson County\tH1\n72168\t5069\tTucker\tAR\tJefferson County\tH1\n71644\t5069\tGrady\tAR\tJefferson County\tH1\n72132\t5069\tRedfield\tAR\tJefferson County\tH1\n72152\t5069\tSherrill\tAR\tJefferson County\tH1\n72830\t5071\tClarksville\tAR\tJohnson County\tH1\n72821\t5071\tAltus\tAR\tJohnson County\tH1\n72845\t5071\tKnoxville\tAR\tJohnson County\tH1\n72839\t5071\tHagarville\tAR\tJohnson County\tH1\n72840\t5071\tHartman\tAR\tJohnson County\tH1\n72847\t5071\tLondon\tAR\tJohnson County\tH1\n72752\t5071\tPettigrew\tAR\tJohnson County\tH1\n72949\t5071\tOzark\tAR\tJohnson County\tH1\n72832\t5071\tCoal hill\tAR\tJohnson County\tH1\n72852\t5071\tOark\tAR\tJohnson County\tH1\n72846\t5071\tLamar\tAR\tJohnson County\tH1\n72854\t5071\tOzone\tAR\tJohnson County\tH1\n71861\t5073\tTaylor\tAR\tLafayette County\tH1\n71827\t5073\tBuckner\tAR\tLafayette County\tH1\n71826\t5073\tBradley\tAR\tLafayette County\tH1\n71860\t5073\tStamps\tAR\tLafayette County\tH1\n71845\t5073\tLewisville\tAR\tLafayette County\tH1\n72440\t5075\tLynn\tAR\tLawrence County\tH1\n72469\t5075\tStrawberry\tAR\tLawrence County\tH1\n72466\t5075\tSmithville\tAR\tLawrence County\tH1\n72416\t5075\tBono\tAR\tLawrence County\tH1\n72445\t5075\tMinturn\tAR\tLawrence County\tH1\n72459\t5075\tRavenden\tAR\tLawrence County\tH1\n72476\t5075\tWalnut ridge\tAR\tLawrence County\tH1\n72433\t5075\tHoxie\tAR\tLawrence County\tH1\n72434\t5075\tImboden\tAR\tLawrence County\tH1\n72572\t5075\tSaffell\tAR\tLawrence County\tH1\n72465\t5075\tSedgwick\tAR\tLawrence County\tH1\n72415\t5075\tBlack rock\tAR\tLawrence County\tH1\n72410\t5075\tAlicia\tAR\tLawrence County\tH1\n72482\t5075\tWilliford\tAR\tLawrence County\tH1\n72457\t5075\tPortia\tAR\tLawrence County\tH1\n72458\t5075\tPowhatan\tAR\tLawrence County\tH1\n72366\t5077\tMarvell\tAR\tLee County\tH1\n72355\t5077\tLexa\tAR\tLee County\tH1\n72360\t5077\tMarianna\tAR\tLee County\tH1\n72320\t5077\tBrickeys\tAR\tLee County\tH1\n72374\t5077\tPoplar grove\tAR\tLee County\tH1\n72335\t5077\tForrest city\tAR\tLee County\tH1\n72348\t5077\tHughes\tAR\tLee County\tH1\n72341\t5077\tHaynes\tAR\tLee County\tH1\n72368\t5077\tMoro\tAR\tLee County\tH1\n72372\t5077\tPalestine\tAR\tLee County\tH1\n72352\t5077\tLa grange\tAR\tLee County\tH1\n72311\t5077\tAubrey\tAR\tLee County\tH1\n71603\t5079\tPine bluff\tAR\tLincoln County\tH1\n71655\t5079\tMonticello\tAR\tLincoln County\tH1\n71639\t5079\tDumas\tAR\tLincoln County\tH1\n71678\t5079\tYorktown\tAR\tLincoln County\tH1\n71667\t5079\tStar city\tAR\tLincoln County\tH1\n71601\t5079\tPine bluff\tAR\tLincoln County\tH1\n71675\t5079\tWilmar\tAR\tLincoln County\tH1\n71644\t5079\tGrady\tAR\tLincoln County\tH1\n71643\t5079\tGould\tAR\tLincoln County\tH1\n71853\t5081\tOgden\tAR\tLittle River County\tH1\n71865\t5081\tWilton\tAR\tLittle River County\tH1\n71836\t5081\tForeman\tAR\tLittle River County\tH1\n71820\t5081\tAlleene\tAR\tLittle River County\tH1\n71866\t5081\tWinthrop\tAR\tLittle River County\tH1\n71822\t5081\tAshdown\tAR\tLittle River County\tH1\n72933\t5083\tCharleston\tAR\tLogan County\tH1\n72928\t5083\tBranch\tAR\tLogan County\tH1\n72943\t5083\tMagazine\tAR\tLogan County\tH1\n72851\t5083\tNew blaine\tAR\tLogan County\tH1\n72927\t5083\tBooneville\tAR\tLogan County\tH1\n72842\t5083\tHavana\tAR\tLogan County\tH1\n72951\t5083\tRatcliff\tAR\tLogan County\tH1\n72865\t5083\tSubiaco\tAR\tLogan County\tH1\n72949\t5083\tOzark\tAR\tLogan County\tH1\n72835\t5083\tDelaware\tAR\tLogan County\tH1\n72834\t5083\tDardanelle\tAR\tLogan County\tH1\n72863\t5083\tScranton\tAR\tLogan County\tH1\n72855\t5083\tParis\tAR\tLogan County\tH1\n72826\t5083\tBlue mountain\tAR\tLogan County\tH1\n72037\t5085\tCoy\tAR\tLonoke County\tH1\n72086\t5085\tLonoke\tAR\tLonoke County\tH1\n72023\t5085\tCabot\tAR\tLonoke County\tH1\n72072\t5085\tHumnoke\tAR\tLonoke County\tH1\n72046\t5085\tEngland\tAR\tLonoke County\tH1\n72142\t5085\tScott\tAR\tLonoke County\tH1\n72076\t5085\tJacksonville\tAR\tLonoke County\tH1\n72160\t5085\tStuttgart\tAR\tLonoke County\tH1\n72083\t5085\tKeo\tAR\tLonoke County\tH1\n72024\t5085\tCarlisle\tAR\tLonoke County\tH1\n72173\t5085\tVilonia\tAR\tLonoke County\tH1\n72007\t5085\tAustin\tAR\tLonoke County\tH1\n72176\t5085\tWard\tAR\tLonoke County\tH1\n72064\t5085\tHazen\tAR\tLonoke County\tH1\n72703\t5087\tFayetteville\tAR\tMadison County\tH1\n72740\t5087\tHuntsville\tAR\tMadison County\tH1\n72773\t5087\tWesley\tAR\tMadison County\tH1\n72632\t5087\tEureka springs\tAR\tMadison County\tH1\n72760\t5087\tSaint paul\tAR\tMadison County\tH1\n72727\t5087\tElkins\tAR\tMadison County\tH1\n72756\t5087\tRogers\tAR\tMadison County\tH1\n72959\t5087\tWinslow\tAR\tMadison County\tH1\n72738\t5087\tHindsville\tAR\tMadison County\tH1\n72721\t5087\tCombs\tAR\tMadison County\tH1\n72752\t5087\tPettigrew\tAR\tMadison County\tH1\n72852\t5087\tOark\tAR\tMadison County\tH1\n72742\t5087\tKingston\tAR\tMadison County\tH1\n72776\t5087\tWitter\tAR\tMadison County\tH1\n72661\t5089\tOakland\tAR\tMarion County\tH1\n72601\t5089\tHarrison\tAR\tMarion County\tH1\n72619\t5089\tBull shoals\tAR\tMarion County\tH1\n72668\t5089\tPeel\tAR\tMarion County\tH1\n72634\t5089\tFlippin\tAR\tMarion County\tH1\n72675\t5089\tSaint joe\tAR\tMarion County\tH1\n72633\t5089\tEverton\tAR\tMarion County\tH1\n72677\t5089\tSummit\tAR\tMarion County\tH1\n72653\t5089\tMountain home\tAR\tMarion County\tH1\n72687\t5089\tYellville\tAR\tMarion County\tH1\n72644\t5089\tLead hill\tAR\tMarion County\tH1\n72682\t5089\tValley springs\tAR\tMarion County\tH1\n72672\t5089\tPyatt\tAR\tMarion County\tH1\n71834\t5091\tDoddridge\tAR\tMiller County\tH1\n71854\t5091\tTexarkana\tAR\tMiller County\tH1\n71840\t5091\tGenoa\tAR\tMiller County\tH1\n71837\t5091\tFouke\tAR\tMiller County\tH1\n71839\t5091\tGarland city\tAR\tMiller County\tH1\n72330\t5093\tDyess\tAR\tMississippi County\tH1\n72438\t5093\tLeachville\tAR\tMississippi County\tH1\n72329\t5093\tDriver\tAR\tMississippi County\tH1\n72321\t5093\tBurdette\tAR\tMississippi County\tH1\n72370\t5093\tOsceola\tAR\tMississippi County\tH1\n72391\t5093\tWest ridge\tAR\tMississippi County\tH1\n72426\t5093\tDell\tAR\tMississippi County\tH1\n72315\t5093\tBlytheville\tAR\tMississippi County\tH1\n72354\t5093\tLepanto\tAR\tMississippi County\tH1\n72428\t5093\tEtowah\tAR\tMississippi County\tH1\n72310\t5093\tArmorel\tAR\tMississippi County\tH1\n72358\t5093\tLuxora\tAR\tMississippi County\tH1\n72386\t5093\tTyronza\tAR\tMississippi County\tH1\n72338\t5093\tFrenchmans bayou\tAR\tMississippi County\tH1\n72419\t5093\tCaraway\tAR\tMississippi County\tH1\n72351\t5093\tKeiser\tAR\tMississippi County\tH1\n72316\t5093\tBlytheville\tAR\tMississippi County\tH1\n72350\t5093\tJoiner\tAR\tMississippi County\tH1\n72395\t5093\tWilson\tAR\tMississippi County\tH1\n72442\t5093\tManila\tAR\tMississippi County\tH1\n72313\t5093\tBassett\tAR\tMississippi County\tH1\n72021\t5095\tBrinkley\tAR\tMonroe County\tH1\n72366\t5095\tMarvell\tAR\tMonroe County\tH1\n72134\t5095\tRoe\tAR\tMonroe County\tH1\n72108\t5095\tMonroe\tAR\tMonroe County\tH1\n72392\t5095\tWheatley\tAR\tMonroe County\tH1\n72029\t5095\tClarendon\tAR\tMonroe County\tH1\n72368\t5095\tMoro\tAR\tMonroe County\tH1\n72069\t5095\tHolly grove\tAR\tMonroe County\tH1\n72036\t5095\tCotton plant\tAR\tMonroe 
